vi "Find current users index.vi"(4 "User access cluster":T1 {"Expire sec" format="%.2f"}, 5 "User array":T3 {"Expire sec" format="%.2f"}) -> (1 "index":i32)   [LabVIEW 2013]
doc: "Searches through the user array for the element with the same User ID as in User Access Cluster and returns in \"Index\". If not found, returns -1."
uses:
  User Access Type defs/User access cluster array.ctl
  User Access Type defs/User access cluster.ctl
  User Access Type defs/Security level U8.ctl
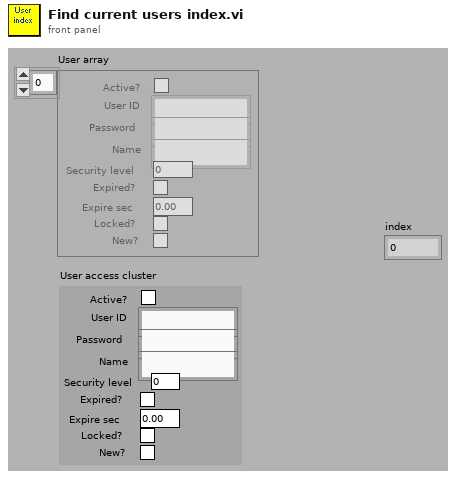
[diagram p1: front panel]
types:
  T1 = typedef "User access cluster.ctl" = cluster{"Active?":bool, "User ID":string, "Password":string, "Name":string, "Security level":T2, "Expired?":bool, "Expire sec":dbl, "Locked?":bool, "New?":bool}
  T2 = typedef "Security level U8.ctl" = u8
  T3 = typedef "User access cluster array.ctl" = T1[]
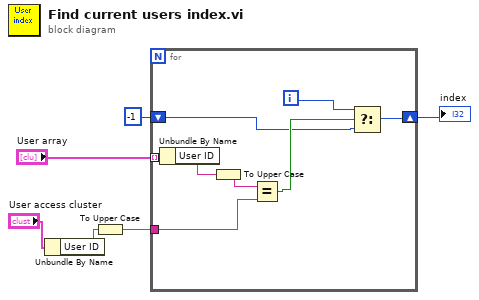
[diagram p0: block diagram]
diagram:
  n1 = Unbundle By Name("User access cluster") -> ("User ID"=w2:string)
  n2 = To Upper Case(1:w2) -> (0:w1:string)
  n3 = for {
    shift-right: [w7] -> w5
    shift-left: -1 ("index") -> [w8]
    tunnel: "User array" -> [w14] mode=indexing
    tunnel: w1 -> [w11]
    i -> [w9]
    n4 = Unbundle By Name(w14) -> ("User ID"=w13:string)
    n5 = To Upper Case(1:w13) -> (0:w12:string)
    n6 = Equal?(x=w12, y=w11) -> (x = y?=w10:bool)
    n7 = Select(t=w9, s=w10, f=w8) -> (s? t:f=w7:i32)
  }
  "index" <- w5
